vi "SplittingStrings.vi"(11 "TEXT":string) -> (1 "Array that contains proper offsets in flash memory":i32[](array[numeric]), 2 "Array that contains proper number of data files in flash memory":i32[](array[numeric]), 3 "Array of 16-signs long strings which will be wrote in flash memory":string[](array[string]))   [LabVIEW 2014]
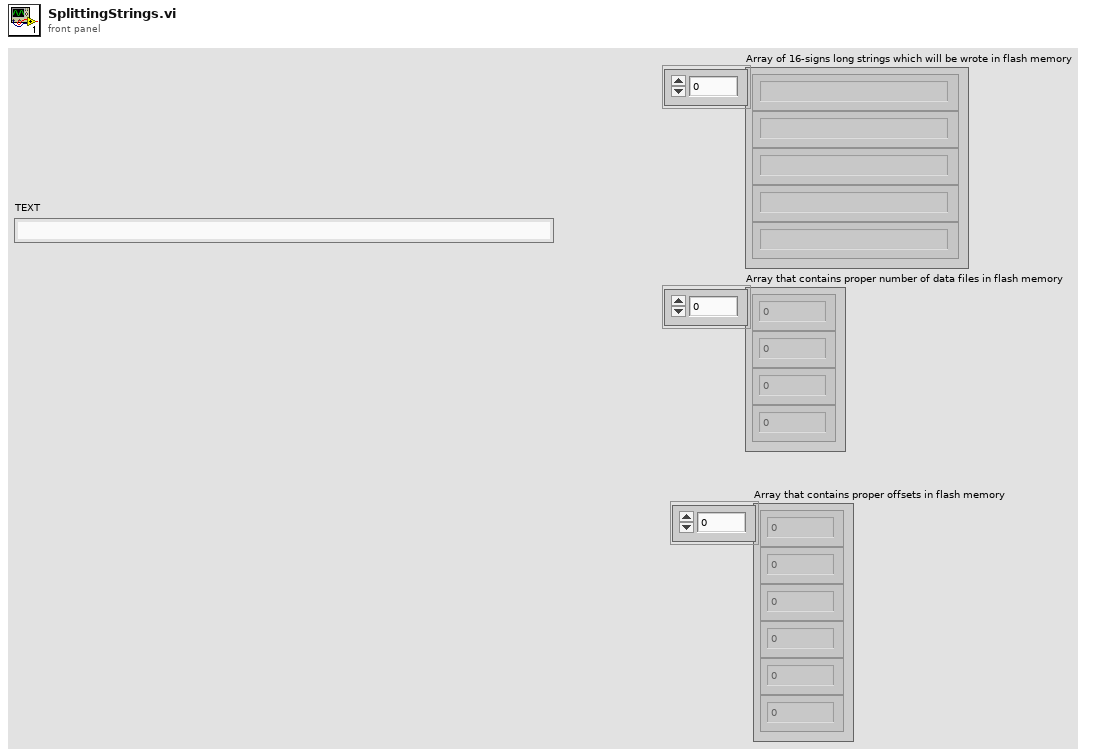
[diagram p1: front panel]
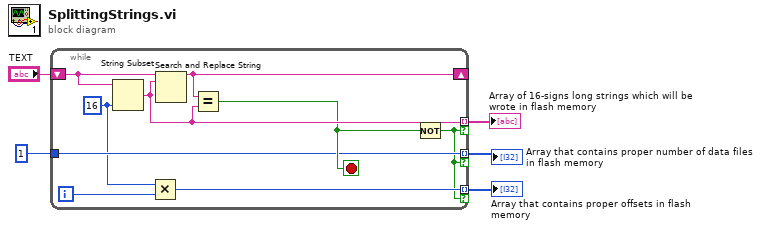
[diagram p0: block diagram]
diagram:
  n1 = while {
    shift-right: [w13] -> _
    shift-left: "TEXT" -> [w14]
    tunnel: [w12] -> w4 mode=indexing if=w6
    tunnel: 1 -> [w10]
    tunnel: [w10] -> w2 mode=indexing if=w6
    tunnel: [w7] -> w1 mode=indexing if=w6
    i -> [w8]
    stop <- w11 stop-if-true
    w9 = 16 ("length (rest)")
    n2 = String Subset(string=w14, length (rest)=w9) -> (substring=w12:string)  [unwired: 1 in]
    n3 = Multiply(x=w9, y=w8) -> (x*y=w7:i32)
    n4 = Search and Replace String(input string=w14, search string=w12) -> (result string=w13:string)  [unwired: 6 in, 3 out]
    n5 = Equal?(x=w13, y=w12) -> (x = y?=w11:bool)
    n6 = Not(x=w11) -> (.not. x?=w6:bool)
  }
  "Array of 16-signs long strings which will be wrote in flash memory" <- w4
  "Array that contains proper number of data files in flash memory" <- w2
  "Array that contains proper offsets in flash memory" <- w1
